vi "Caller.vi"(0 "Subtract in":refnum<class "Subtract.lvclass">, 5 "Sub Panel":refnum<vi>, 7 "State":refnum<user-event>, 9 "Class Data":refnum<user-event>, 11 "Error In":errorcluster) -> (4 "Subtract out":refnum<class "Subtract.lvclass">, 15 "Error Out":errorcluster)   [LabVIEW 2023, in "Subtract.lvclass"]
doc: "The VI asynchronously calls the Operation UI method of the subtraction operation."
uses:
  Subtract.lvclass
  C:/Users/Ancy.Augustin/Downloads/LVOOPS DVR/LVOOPS DVR/Classes/Arithemtic Operation/Arithemetic Operation.lvclass
  Arithemtic Operation/Arithemetic Operation.lvclass
  Operation UI.vi
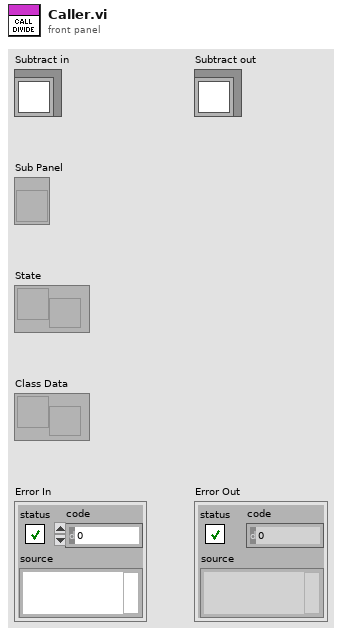
[diagram p1: front panel]
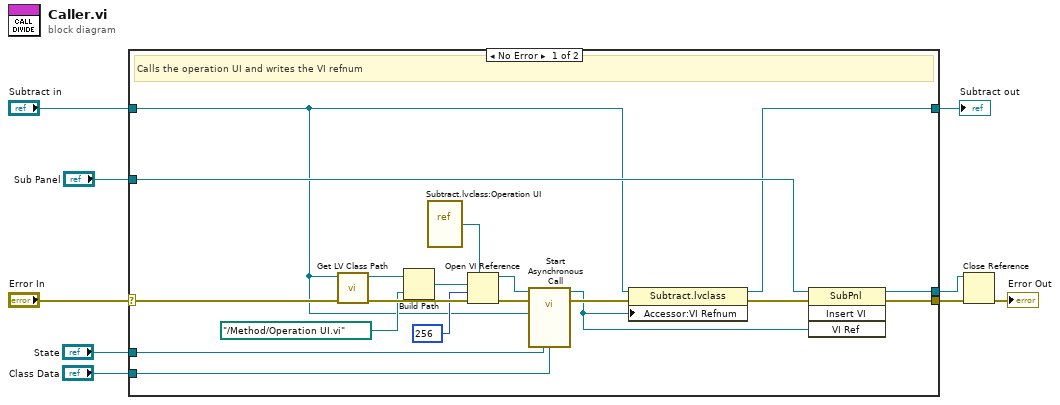
[diagram p0: block diagram]
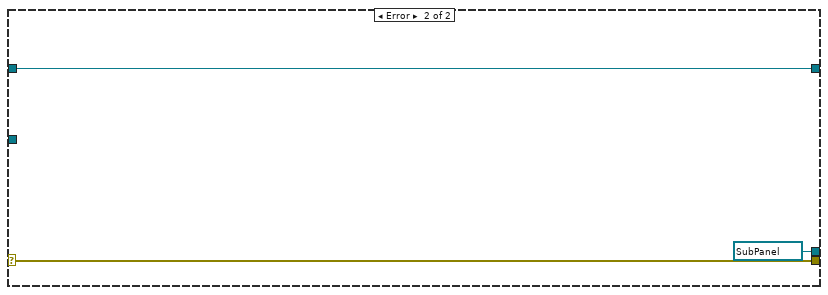
[diagram p2: hidden frame]
diagram:
  n1 = case shown="No Error" "Error In" {
    selector: "Error In" -> [w19 w31]
    tunnel: [w18 w31] -> w8
    tunnel: [w12 w30] -> w6
    tunnel: "Subtract in" -> [w10 w30]
    tunnel: "State" -> [w17 _]
    tunnel: "Class Data" -> [w16 _]
    tunnel: "Sub Panel" -> [w15 _]
    tunnel: [w11 refnum<vi> refnum ("Sub Panel")] -> w1
    frame No Error {
      # "Calls the operation UI and writes the VI refnum"
      n2 = call <vilib>:"Get LV Class Path.vi"("error in (no error)"=w19, "object"=w10) -> ("error out"=w28:errorcluster, "class path"=w27:path)  [unwired: 8 in]
      n3 = Build Path(base path=w27, name or relative path=path "../Method/Operation UI.vi") -> (appended path=w24:path)
      n4 = vi-ref "Subtract.lvclass:Operation UI.vi"() -> (w20:refnum<vi>)
      n5 = Open VI Reference(type specifier VI Refnum (for type only)=w20, vi path=w24, options=256, error in (no error)=w28) -> (vi reference=w23:refnum<vi>, error out=w25:errorcluster)  [unwired: 2 in]
      n6 = call-by-ref "Start Asynchronous Call"(reference=w23, error in=w25, "Subtract in"=w10, "user event out 2"=w17, "user event out"=w16) -> (reference out=w13:refnum<vi>, error out=w22:errorcluster)  [unwired: 10 in, 3 out]
      n7 = property class="Subtract.lvclass"(reference=w10, error in=w22, "Accessor:VI Refnum"=w13) -> (reference out=w12:refnum<class "Subtract.lvclass">, error out=w14:errorcluster)
      n8 = invoke on="Invoke Node" class="SubPnl" method="Insert VI"(reference=w15, error in=w14, "VI Ref"=w13) -> (reference out=w11:refnum<vi>, error out=w18:errorcluster)  [unwired: 1 in, 2 out]
    }
    frame Error {
    }
  }
  "Subtract out" <- w6
  n9 = Close Reference(reference=w1, error in (no error)=w8) -> (error out=→"Error Out":errorcluster)
